vi "Load Scale And Calibration from file.vi"(8 "error in (no error)":errorcluster, 10 "polynomial order":i32=5, 11 "appended path":path) -> (0 "error out":errorcluster, 1 "all rows":dbl[][](array[numeric]), 2 "intercept":dbl, 3 "slope":dbl, 4 "Measurement":dbl[](array[numeric]), 5 "Polynomial Coefficients":dbl[](array[numeric]) format="%#_15g", 6 "Physical Units":dbl[](array[numeric]))   [LabVIEW 2017]
uses:
  <vilib>/Utility/file.llb/Read From Spreadsheet File (DBL).vi
  <vilib>/Analysis/NI_AALPro.lvlib
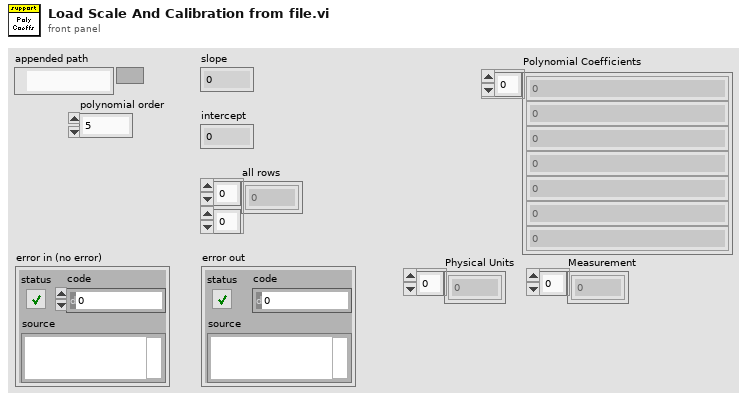
[diagram p1: front panel]
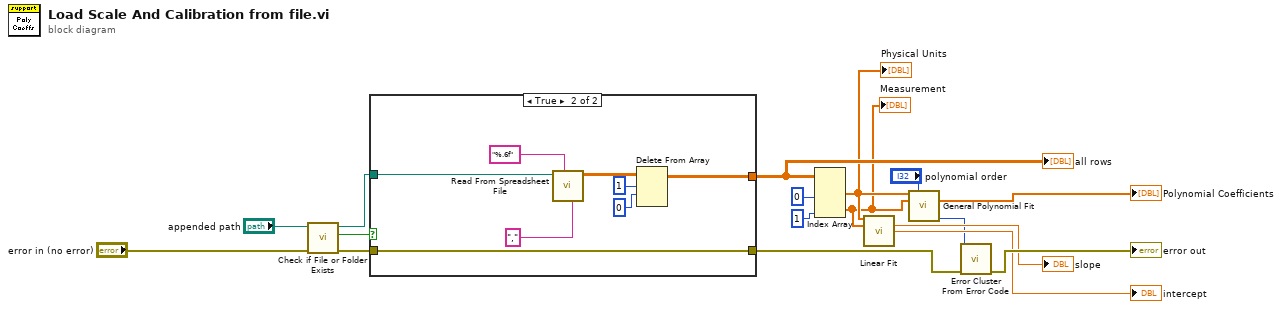
[diagram p0: block diagram]
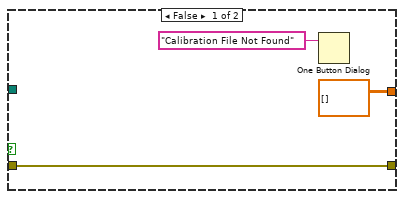
[diagram p2: hidden frame]
diagram:
  n1 = call <vilib>:"Check if File or Folder Exists.vi"("error in (no error)"="error in (no error)", "path"="appended path") -> ("error out"=w9:errorcluster, "file or folder exists?"=w10:bool, "dup path"=w11:path)  [unwired: 7 in]
  n2 = case shown="True" w10 {
    tunnel: w9 -> [w20 w28]
    tunnel: [w20 w28] -> w1
    tunnel: w11 -> [_ w27]
    tunnel: [dbl[][] [] ("all rows") w21] -> w17
    frame False {
      n3 = One Button Dialog(message="Calibration File Not Found") -> ()  [unwired: 1 in, 1 out]
    }
    frame True {
      n4 = call-poly <vilib>:"Read From Spreadsheet File.vi"("delimiter (\\t)"="," ("delimiter (\\t)"), "format (%.3f)"="%.6f", "file path (dialog if empty)"=w27) -> ("all rows"=w24:dbl[][])  [unwired: 4 in, 4 out]
      n5 = Delete From Array(array=w24, length=1, index (row)=0) -> (array with subset deleted=w21:dbl[][])  [unwired: 1 in, 1 out]
    }
  }
  "all rows" <- w17
  n6 = Index Array(array=w17, index (col) #1=0 ("disabled index (col)"), index (col) #2=1 ("index (col)")) -> (element #1=w4:dbl[], element #2=w3:dbl[])  [unwired: 2 in]
  "Physical Units" <- w4
  "Measurement" <- w3
  n7 = call <vilib>:"Linear Fit.vi"("Y"=w4, "X"=w3) -> ("slope"=→"slope":dbl, "intercept"=→"intercept":dbl)  [unwired: 9 in, 3 out]
  n8 = call <vilib>:"General Polynomial Fit.vi"("Y"=w4, "polynomial order"="polynomial order", "X"=w3) -> ("Polynomial Coefficients"=→"Polynomial Coefficients":dbl[], "error"=w2:i32)  [unwired: 9 in, 2 out]
  n9 = call <vilib>:"Error Cluster From Error Code.vi"("error in (no error)"=w1, "error code (0)"=w2) -> ("error out"=→"error out":errorcluster)  [unwired: 7 in]
